vi "Replace Line.vi"(8 "error in":errorcluster, 9 "New Line":T1={"channel"=refnum, "XNET Signal"="CANEventSignal1\nNIXNET_example.CAN_Cluster"}, 10 "Line Name":string, 11 "J1939 configuration in":refnum<class "J1939 configuration.lvclass">) -> (0 "error out":errorcluster, 2 "Old Line":T1={"channel"=refnum, "XNET Signal"="CANEventSignal1\nNIXNET_example.CAN_Cluster"}, 3 "J1939 configuration out":refnum<class "J1939 configuration.lvclass">)   [LabVIEW 2014, in "J1939 configuration.lvclass"]
doc: "Replaces a line identified by name with a new line."
uses:
  J1939 configuration.lvclass
  Line.ctl
  <vilib>/NI/Tag Bus Module Framework/channel/TBM channel.lvclass
  J1939 configuration.lvclass/J1939 configuration.ctl
  <vilib>/NI/Tag Bus Module Framework/module configuration/TBM module configuration.lvclass
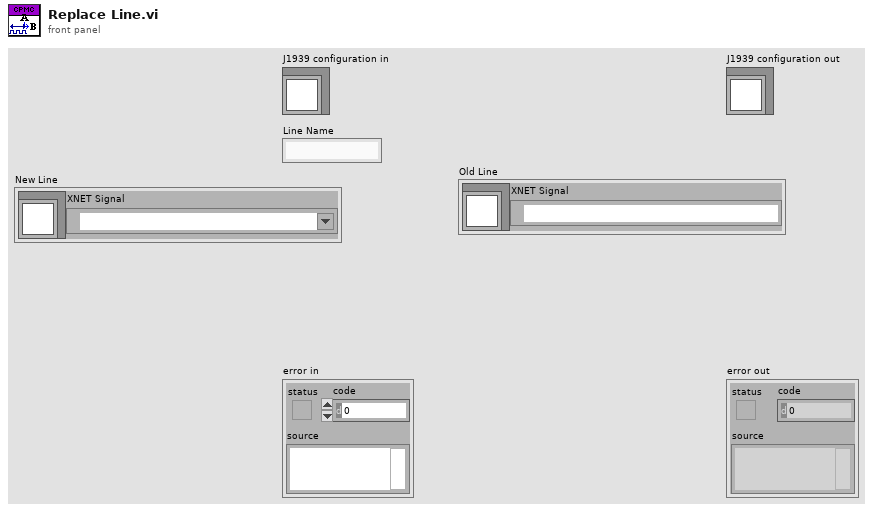
[diagram p1: front panel]
types:
  T1 = typedef "J1939 configuration.lvclass/Line.ctl" = cluster{"channel":refnum<class "TBM channel.lvclass">, "XNET Signal":refnum<k21>}
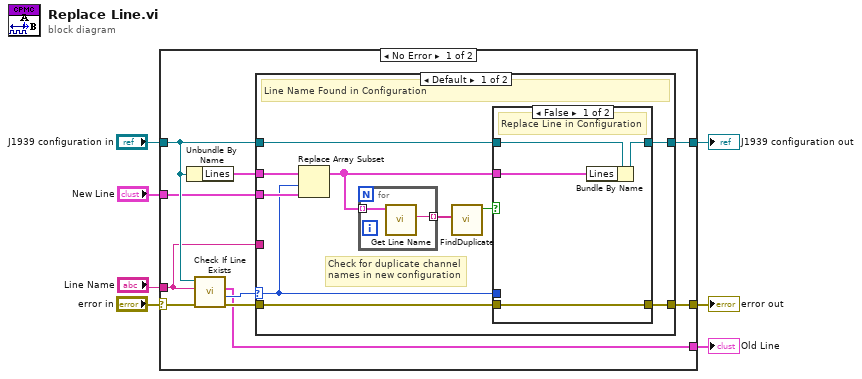
[diagram p0: block diagram]
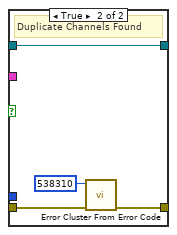
[diagram p2: hidden frame]
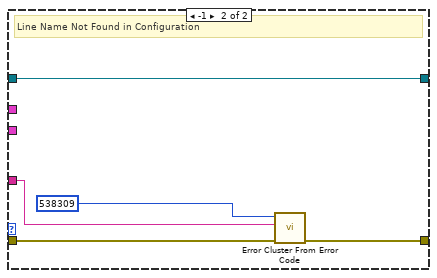
[diagram p3: hidden frame]
diagram:
  n1 = case shown="No Error" "error in" {
    selector: "error in" -> [w10 w44]
    tunnel: [w16 w44] -> w6
    tunnel: [w17 w43] -> w4
    tunnel: "J1939 configuration in" -> [w15 w43]
    tunnel: "Line Name" -> [w14 _]
    tunnel: "New Line" -> [w12 _]
    tunnel: [w8 _] -> w1
    frame No Error {
      n2 = Unbundle By Name(w15) -> ("Lines"=w11:T1[])
      n3 = call-dynamic "Check If Line Exists.vi"("error in"=w10, "Name to Locate"=w14, "J1939 configuration in"=w15) -> ("error out"=w9:errorcluster, "Index"=w13:i32, "Line out"=w8:T1)  [unwired: 4 in, 2 out]
      n4 = case shown="Default" w13 {
        selector: w13 -> [w20 _]
        tunnel: w15 -> [w27 w42]
        tunnel: [w26 w42] -> w17
        tunnel: w11 -> [w22 _]
        tunnel: w12 -> [w21 _]
        tunnel: w14 -> [_ w40]
        tunnel: w9 -> [w24 w39]
        tunnel: [w18 w38] -> w16
        frame Default {
          # "Check for duplicate channel names in new configuration"
          # "Line Name Found in Configuration"
          n5 = Replace Array Subset(array=w22, new element=w21, index=w20) -> (w19:T1[])
          n6 = for {
            tunnel: w19 -> [w29] mode=indexing
            tunnel: [w28] -> w25 mode=indexing
            n7 = call "Get Line Name.vi"("Line in"=w29) -> ("Name"=w28:string)  [unwired: 8 in, 2 out]
          }
          n8 = call <vilib>:"FindDuplicate.vi"("Array"=w25) -> ("Duplicate"=w23:bool)  [unwired: 8 in, 2 out]
          n9 = case shown="False" w23 {
            tunnel: w27 -> [w33 w37]
            tunnel: [w32 w37] -> w26
            tunnel: w20 -> [_ _]
            tunnel: w24 -> [w30 w36]
            tunnel: w19 -> [w31 _]
            tunnel: [w30 w35] -> w18
            frame False {
              # "Replace Line in Configuration"
              n10 = Bundle By Name(cluster=w33, "Lines"=w31) -> (w32:refnum<class "J1939 configuration.lvclass">)
            }
            frame True {
              # "Duplicate Channels Found"
              n11 = call <vilib>:"Error Cluster From Error Code.vi"("error in (no error)"=w36, "error code (0)"=538310) -> ("error out"=w35:errorcluster)  [unwired: 7 in]
            }
          }
        }
        frame -1 {
          # "Line Name Not Found in Configuration"
          n12 = call <vilib>:"Error Cluster From Error Code.vi"("error in (no error)"=w39, "error message (\"\")"=w40, "error code (0)"=538309) -> ("error out"=w38:errorcluster)  [unwired: 6 in]
        }
      }
    }
    frame Error {
    }
  }
  "error out" <- w6
  "J1939 configuration out" <- w4
  "Old Line" <- w1
